vi "FTW-Socket-Ask.vi"(0 "FTW Socket":refnum<class "FTW-Socket.lvclass">, 5 "Request":string, 7 "Receive Timeout":i32=100 format="%dmsec", 9 "Send Timeout":i32 format="%dmsec", 11 "error in":errorcluster) -> (4 "FTW Socket out":refnum<class "FTW-Socket.lvclass">, 6 "Response":string, 8 "Timed out?":bool, 10 "Roundtrip Time":dbl format="%.4psec", 15 "error out":errorcluster)   [LabVIEW 2013, in "FTW-Socket.lvclass"]
uses:
  FTW-Socket.lvclass
  FTW-Socket.lvclass/FTW-Socket.ctl
panel:
  # "Inputs"
  # "Outputs"
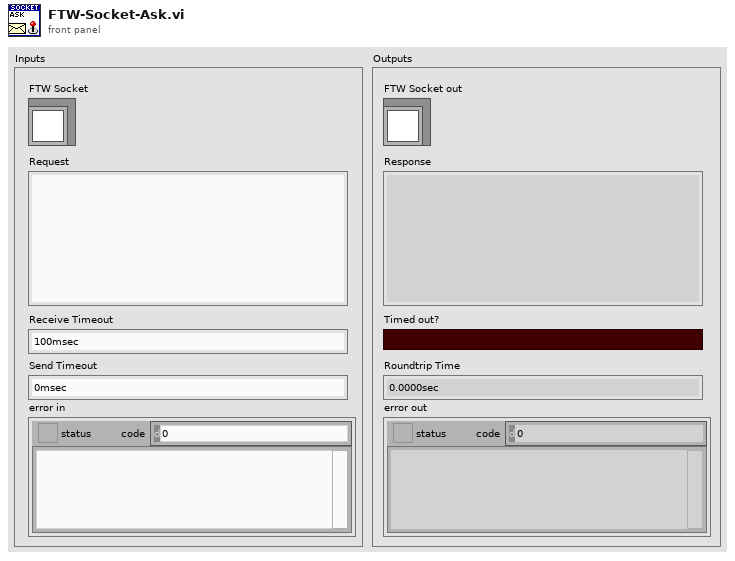
[diagram p1: front panel]
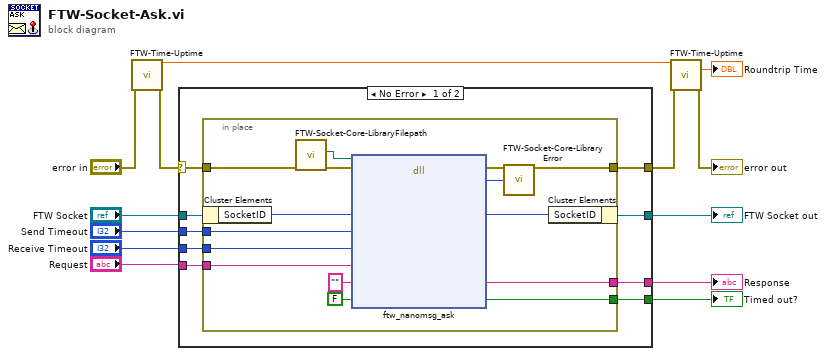
[diagram p0: block diagram]
diagram:
  n1 = call "FTW-Time-Uptime.vi"("error in"="error in") -> ("Current Uptime"=w2:dbl, "error out"=w5:errorcluster)  [unwired: 12 in, 1 out]
  n2 = case shown="No Error" w5 {
    selector: w5 -> [w18 w38]
    tunnel: "FTW Socket" -> [w22 w39]
    tunnel: "Request" -> [w21 _]
    tunnel: [w20 w38] -> w3
    tunnel: [w19 w39] -> w10
    tunnel: "Receive Timeout" -> [w17 _]
    tunnel: [w15 _] -> w9
    tunnel: "Send Timeout" -> [w16 _]
    tunnel: [w14 _] -> w7
    frame No Error {
      n3 = in-place {
        in-place-border: w18 -> [w37]
        in-place-border: [w33] -> w20
        in-place-border: [w32] -> w15
        in-place-border: w16 -> [w29]
        in-place-border: w17 -> [w28]
        in-place-border: w21 -> [w26]
        in-place-border: [w24] -> w14
        n4 = in-place-cluster #1(w22) -> ("SocketID"=w35:i64)
        n5 = call "FTW-Socket-Core-LibraryFilepath.vi"("error in"=w37) -> ("error out"=w30:errorcluster, "Library Filepath"=w31:path)  [unwired: 8 in, 1 out]
        n6 = dll-call lib="?" fn="ftw_nanomsg_ask"(path in=w31, error in=w30, "SocketID"=w35, "Send Timeout"=w29, "Recv Timeout"=w28, "Request"=w26, "Response"="", "Timed out?"=FALSE) -> (error out=w36:errorcluster, "Return Value"=w27:i64, "SocketID"=w34:i64, "Response"=w32:string, "Timed out?"=w24:bool)  [unwired: 6 in, 1 out]
        n7 = call "FTW-Socket-Core-LibraryError.vi"("error in"=w36, "Return Value"=w27) -> ("error out"=w33:errorcluster)  [unwired: 13 in]
        n8 = in-place-cluster #1("SocketID"=w34) -> (w19:refnum<class "FTW-Socket.lvclass">)
      }
    }
    frame Error {
    }
  }
  "FTW Socket out" <- w10
  "Timed out?" <- w7
  "Response" <- w9
  n9 = call "FTW-Time-Uptime.vi"("Previous Uptime"=w2, "error in"=w3) -> ("Elapsed Time"=→"Roundtrip Time":dbl, "error out"=→"error out":errorcluster)  [unwired: 11 in, 1 out]
